vi "maxint_backup.vi"() -> ()   [LabVIEW 2020]
uses:
  <vilib>/userdefined/High Color/IMAQdx.ctl
  C:/Users/lenovo/source/repos/MSMQ_try/how/bin/Release/how.dll
  source/repos/MSMQ_try/how/bin/Release/how.dll
  C:/Users/lenovo/source/repos/MSMQ_try/Calculator/bin/Debug/Calculator.dll
  source/repos/MSMQ_try/Calculator/bin/Debug/Calculator.dll
  C:/Users/lenovo/source/repos/MSMQ_try/Pallete_maker/bin/Debug/Pallete_maker.dll
  source/repos/MSMQ_try/Pallete_maker/bin/Debug/Pallete_maker.dll
  C:/Users/lenovo/source/repos/MSMQ_try/MIrror_x64/bin/Debug/MIrror_x64.dll
  source/repos/MSMQ_try/MIrror_x64/bin/Debug/MIrror_x64.dll
  <vilib>/vision/driver/NI_Vision_Acquisition_Software.lvlib
  <resource>/objmgr/imaqdx.rc
  source/repos/cont2019/x64/Release/Image_processing.dll
panel:
  in  "log_data":i32=1
  in  "Exposure time":dbl=5000.0
  out "Waveform Chart":dbl(graph)
  in  "amplitude_limit":dbl=0.1
  in  "phi_v":dbl
  in  "phi_g":dbl=1.6
  in  "phi_p":dbl=1.2
  in  "vel_limit":dbl=0.4
  in  "init_zero":bool
  in  "level":dbl
  in  "factor":dbl
  out "Waveform Graph 2":dbl[](graph)
  in  "gamma":dbl=0.1
  in  "stop":bool
  in  "cam":bool
  out "mirror params":string
  in  "DM":bool
  out "Iterations":i32
  out "global_best_value":dbl
  out "Waveform Graph":dbl[](graph)
  out "Image":T1(plugin-control)
  out "metrics":dbl[](array[numeric])
  out "Numeric":dbl
  out "Exposure time":dbl
  out "najor":bool
  out "width":i32
  out "height":i32
  out "Intensity Graph":u8[][](graph)
  in  "Session In":T2="cam2"
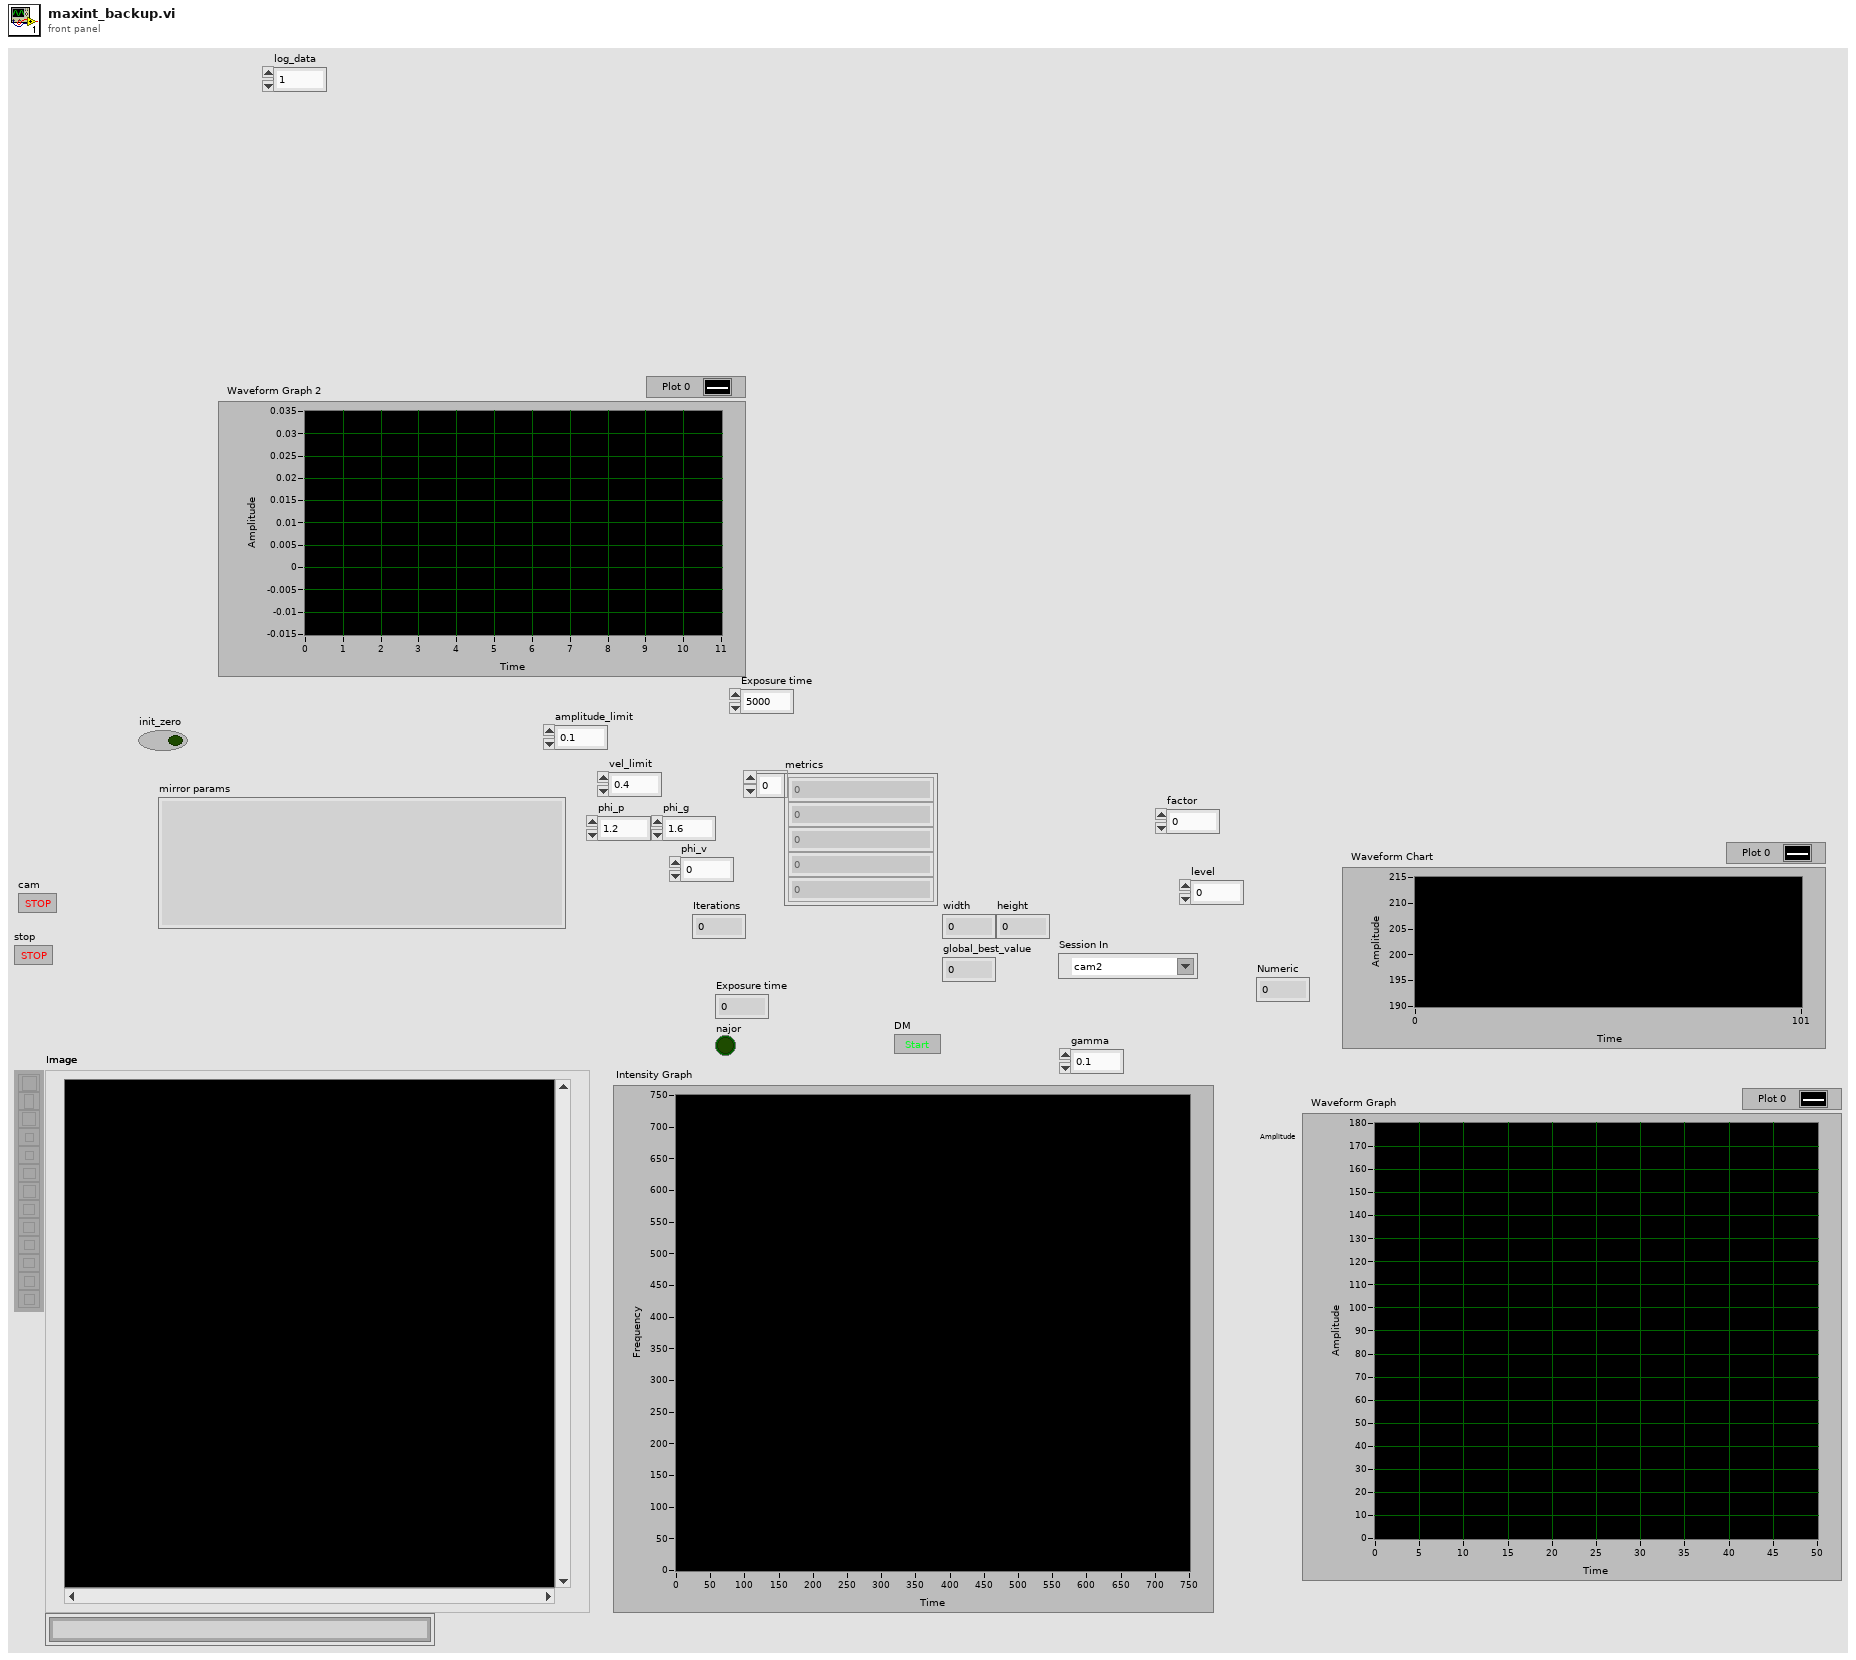
[diagram p1: front panel]
types:
  T1 = typedef "IMAQ Image.ctl" = refnum<image>
  T2 = typedef "IMAQdx.ctl" = refnum<k21>
  T3 = enum32{"Gray", "Binary", "Gradient", "Rainbow", "Temperature"}
  T4 = cluster{"Global Rectangle":i32[], "Contours":cluster{"Contour Type":u32, "ROI Type":u32, "Points":i32[]}[]}
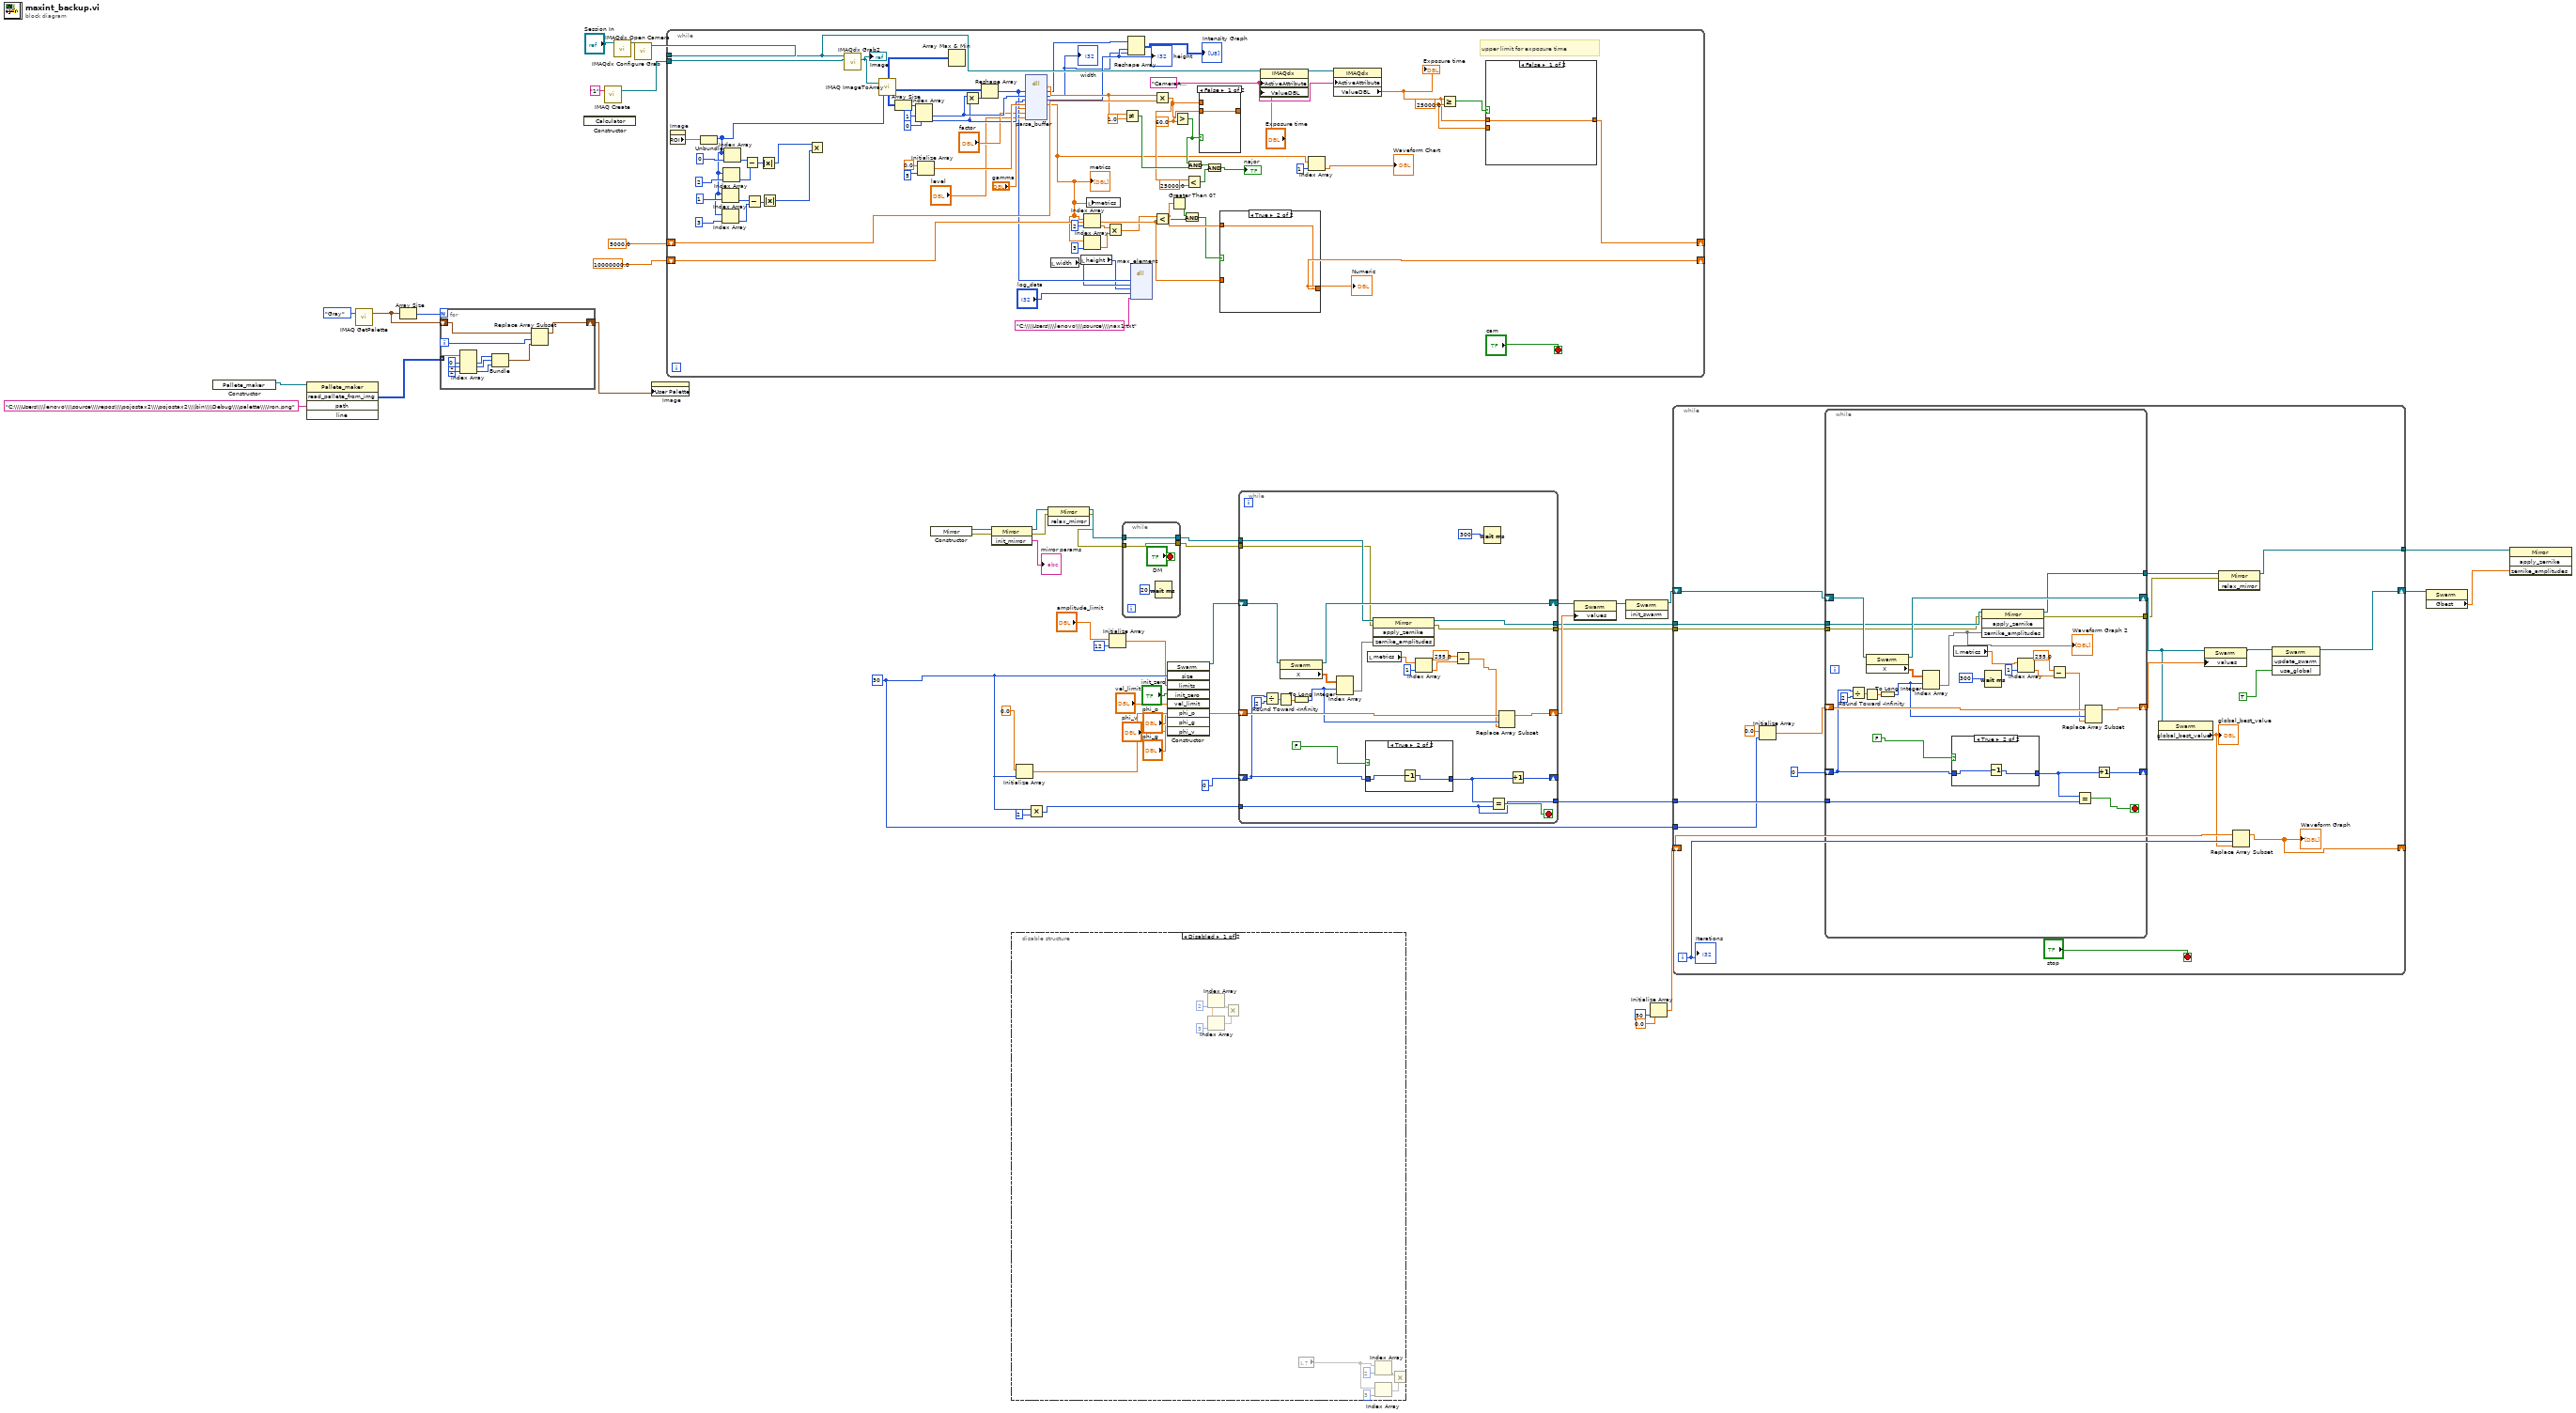
[diagram p0: block diagram]
diagram:
  w26 = 30 ("size")
  n1 = constructor class="Pallete_maker"() -> (reference out=w39:refnum<k24>)  [unwired: 3 in, 2 out]
  n2 = invoke class="Pallete_maker" method="read_pallete_from_img"(reference=w39, "path"="C:\\\\Users\\\\lenovo\\\\source\\\\repos\\\\pojostax2\\\\pojostax2\\\\bin\\\\Debug\\\\palette\\\\Iron.png") -> ("read_pallete_from_img"=w40:u8[][])  [unwired: 3 in, 4 out]
  n3 = call "IMAQ GetPalette"("Palette Number (gray)"=T3."Gray") -> ("Color Palette"=w42:cluster{"Red":u8, "Green":u8, "Blue":u8}[])  [unwired: 4 in, 1 out]
  n4 = Array Size(array=w42) -> (size(s)=w43:i32)
  n5 = for {
    N: w43 -> [_]
    shift-right: [w52] -> w38
    shift-left: w42 -> [w54]
    tunnel: w40 -> [w62] mode=indexing
    i -> [w53]
    n6 = Index Array(array=w62, index #1=0 ("index"), index #2=1 ("index"), index #3=2 ("index")) -> (element #1=w58:u8, element #2=w57:u8, element #3=w56:u8)
    n7 = Bundle(w58, w57, w56) -> (w55:cluster{u8, u8, u8})  [unwired: 1 in]
    n8 = Replace Array Subset(array=w54, new element=w55, index=w53) -> (w52:cluster{"Red":u8, "Green":u8, "Blue":u8}[])
  }
  n9 = constructor class="Calculator"() -> ()  [unwired: 3 in, 3 out]
  n10 = call "IMAQ Create"("Image Name"="1") -> ("New Image"=w47:T1)  [unwired: 4 in, 1 out]
  n11 = call <vilib>:"IMAQdx Open Camera.vi"("Session In"="Session In") -> ("Session Out"=w49:T2)  [unwired: 9 in, 1 out]
  n12 = call <vilib>:"IMAQdx Configure Grab.vi"("Session In"=w49) -> ("Session Out"=w48:T2)  [unwired: 9 in, 1 out]
  n13 = property on="Image" class="ImageControl"("User Palette"=w38) -> ()  [unwired: 2 in, 2 out]
  n14 = while {
    tunnel: w48 -> [w106]
    tunnel: w47 -> [w133]
    shift-right: [w112] -> _
    shift-left: 10000000.0 -> [w111]
    shift-right: [w101] -> _
    shift-left: 5000.0 -> [w100]
    stop <- "cam" stop-if-true
    w96 = 60.0 ("y")
    w102 = 25000.0 ("y")
    w104 = "CameraAttributes::AcquisitionControl::ExposureTime" ("ValueString")
    # "upper limit for exposure time"
    n15 = property on="Image" class="ImageControl"() -> ("ROI"=w132:T4)  [unwired: 2 in, 2 out]
    n16 = Unbundle(w132) -> ("Global Rectangle"=w121:i32[])  [unwired: 1 out]
    n17 = Index Array(array=w121, index=1) -> (element=w120:i32)
    n18 = Index Array(array=w121, index=3) -> (element=w119:i32)
    n19 = Index Array(array=w121, index=2) -> (element=w122:i32)
    n20 = Index Array(array=w121, index=0) -> (element=w123:i32)
    n21 = Subtract(x=w123, y=w122) -> (x-y=w118:i32)
    n22 = Subtract(x=w120, y=w119) -> (x-y=w117:i32)
    n23 = Absolute Value(x=w118) -> (abs(x)=w92:i32)
    n24 = Absolute Value(x=w117) -> (abs(x)=w93:i32)
    n25 = Multiply(x=w92, y=w93) -> ()  [unwired: 1 out]
    n26 = call <vilib>:"IMAQdx Grab2.vi"("Image In"=w133, "Session In"=w106) -> ("Image Out"=w128:T1)  [unwired: 6 in, 3 out]
    "Image" <- w128
    n27 = call "IMAQ ImageToArray"("Optional Rectangle"=w121, "Image"=w128) -> ("Image Pixels (U8)"=w91:u8[][])  [unwired: 2 in, 4 out]
    n28 = Array Size(array=w91) -> (size(s)=w90:i32[])
    n29 = Index Array(array=w90, index #1=1 ("index"), index #2=0 ("index")) -> (element #1=w86:i32, element #2=w85:i32)
    n30 = Initialize Array(0.0, 5 ("dimension size")) -> (w129:dbl[])
    n31 = Array Max & Min(array=w91) -> ()  [unwired: 4 out]
    n32 = Multiply(x=w86, y=w85) -> (x*y=w87:i32)
    n33 = Reshape Array(w91, w87) -> (w65:u8[])
    n34 = dll-call lib="C:/Users/lenovo/source/repos/cont2019/x64/Release/Image_processing.dll" fn="parse_buffer"("pixel_data"=w65, "width"=w86, "height"=w85, "metrics"=w129, "gamma"="gamma", "factor"="factor", "level"="level") -> ("ET_factor"=w98:dbl, "pixel_data"=w84:u8[], "width"=w82:i32, "height"=w83:i32, "metrics"=w71:dbl[])  [unwired: 6 in, 2 out]
    "metrics" <- w71
    "width" <- w82
    "height" <- w83
    n35 = local read "width"() -> (w64:i32)
    n36 = local read "height"() -> (w63:i32)
    n37 = Index Array(array=w71, index=2) -> (element=w115:dbl)
    n38 = Index Array(array=w71, index=3) -> (element=w116:dbl)
    n39 = local write "metrics"(w71) -> ()
    n40 = Multiply(x=w115, y=w116) -> (x*y=w110:dbl)
    n41 = Not Equal?(x=w98, y=1.0) -> (x != y?=w95:bool)
    n42 = Reshape Array(w84, w83, w82) -> (→"Intensity Graph":u8[][])
    n43 = dll-call lib="C:/Users/lenovo/source/repos/cont2019/x64/Release/Image_processing.dll" fn="max_element"("pixel_data"=w65, "width"=w64, "height"=w63, "log_data"="log_data", "path"="C:\\\\Users\\\\lenovo\\\\source\\\\nax1.txt") -> ()  [unwired: 9 in, 2 out]
    n44 = Multiply(x=w98, y=w100) -> (x*y=w78:dbl)
    n45 = Less?(x=w110, y=w111) -> (x < y?=w108:bool)
    n46 = Greater Than 0?(x=w110) -> (x > 0?=w109:bool)
    n47 = Greater?(x=w78, y=w96) -> (0:w94:bool)
    n48 = And(x=w109, y=w108) -> (x .and. y?=w107:bool)
    n49 = Less?(x=w78, y=25000.0) -> (x < y?=w81:bool)
    n50 = And(x=w94, y=w95) -> (x .and. y?=w80:bool)
    n51 = case shown="False" w94 {
      tunnel: [w134 w135] -> _
      tunnel: w78 -> [_ w135]
      tunnel: w96 -> [w134 _]
      frame False {
      }
      frame True {
      }
    }
    n52 = And(x=w80, y=w81) -> (x .and. y?=→"najor":bool)
    n53 = case shown="True" w107 {
      tunnel: [w138 w139] -> w112
      tunnel: w111 -> [w138 _]
      tunnel: w110 -> [_ w139]
      frame False {
      }
      frame True {
      }
    }
    "Numeric" <- w112
    n54 = property class="IMAQdx"(reference=w106, "ActiveAttribute"=w104, "ValueDBL"="Exposure time") -> (reference out=w105:T2)  [unwired: 1 in, 1 out]
    n55 = Index Array(array=w71, index=1) -> (element=→"Waveform Chart":dbl)
    n56 = property class="IMAQdx"(reference=w105, "ActiveAttribute"=w104) -> ("ValueDBL"=w99:dbl)  [unwired: 1 in, 2 out]
    "Exposure time" <- w99
    n57 = Greater Or Equal?(x=w99, y=w102) -> (x >= y?=w103:bool)
    n58 = case shown="False" w103 {
      tunnel: w102 -> [_ w137]
      tunnel: [w136 w137] -> w101
      tunnel: w99 -> [w136 _]
      frame False {
      }
      frame True {
      }
    }
  }
  n59 = constructor class="Mirror"() -> (reference out=w22:refnum<k24>, error out=w20:errorcluster)  [unwired: 3 in, 1 out]
  n60 = invoke class="Mirror" method="init_mirror"(reference=w22, error in=w20) -> (reference out=w15:refnum<k24>, error out=w14:errorcluster, "init_mirror"=→"mirror params":string)  [unwired: 1 in]
  n61 = disable-structure shown="Disabled" {
    frame Disabled {
      n62 = Index Array(index=3) -> (array=w140:dbl[], element=w144)
      n63 = Index Array(array=w140, index=2) -> (element=w143)
      n64 = Multiply(x=w143, y=w144) -> ()  [unwired: 1 out]
      n65 = local read item#-1() -> (w145)
      n66 = Index Array(array=w145, index=2) -> (element=w148)
      n67 = Index Array(array=w145, index=3) -> (element=w149)
      n68 = Multiply(x=w148, y=w149) -> ()  [unwired: 1 out]
    }
    frame Enabled {
    }
  }
  n69 = Initialize Array(0.0 ("element"), w26) -> (w34:dbl[])
  n70 = Multiply(x=w26, y=2) -> (x*y=w29:i32)
  n71 = invoke class="Mirror" method="relax_mirror"(reference=w15, error in=w14) -> (reference out=w13:refnum<k24>, error out=w12:errorcluster)  [unwired: 1 in, 1 out]
  n72 = Initialize Array("amplitude_limit", 12 ("dimension size")) -> (w4:dbl[])
  n73 = while {
    tunnel: [w152] -> w19
    tunnel: w13 -> [w152]
    tunnel: [w150] -> w18
    tunnel: w12 -> [w150]
    stop <- "DM" stop-if-true
    n74 = Wait (ms)(milliseconds to wait=u32 20) -> ()  [unwired: 1 out]
  }
  n75 = constructor class="Swarm"("size"=w26, "limits"=w4, "init_zero"="init_zero", "vel_limit"="vel_limit", "phi_p"="phi_p", "phi_g"="phi_g", "phi_v"="phi_v") -> (reference out=w35:refnum<k24>)  [unwired: 3 in, 9 out]
  n76 = while {
    shift-right: [w172] -> w32
    shift-left: w34 -> [w173]
    shift-right: [w170] -> w33
    shift-left: w35 -> [w179]
    shift-right: [w169] -> _
    shift-left: 0 -> [w167]
    tunnel: w29 -> [w165]
    tunnel: [w165] -> w27
    tunnel: w19 -> [w164]
    tunnel: w18 -> [w162]
    tunnel: [w161] -> w17
    tunnel: [w160] -> w16
    stop <- w168 stop-if-true
    n77 = Divide(x=w167, y=2) -> (x/y=w177:dbl)
    n78 = Round Toward -Infinity(1:w177) -> (0:w176:dbl)
    n79 = property class="Swarm"(reference=w179) -> (reference out=w170:refnum<k24>, "X"=w175:dbl[][])  [unwired: 1 in, 1 out]
    n80 = To Long Integer(number=w176) -> (32bit integer=w171:i32)
    n81 = Index Array(array=w175, index (row)=w171) -> (element=w163:dbl[])  [unwired: 1 in]
    n82 = case shown="True" FALSE {
      tunnel: w167 -> [w180 w182]
      tunnel: [w180 w181] -> w166
      frame False {
      }
      frame True {
        n83 = Decrement(x=w182) -> (x-1=w181:i32)
      }
    }
    n84 = local read "metrics"() -> (w159:dbl[])
    n85 = invoke class="Mirror" method="apply_zernike"(reference=w164, error in=w162, "zernike_amplitudes"=w163) -> (reference out=w161:refnum<k24>, error out=w160:errorcluster)  [unwired: 1 in, 2 out]
    n86 = Index Array(array=w159, index=1) -> (element=w157:dbl)
    n87 = Subtract(x=255.0, y=w157) -> (x-y=w155:dbl)
    n88 = Wait (ms)(milliseconds to wait=u32 300) -> ()  [unwired: 1 out]
    n89 = Equal?(x=w166, y=w165) -> (x = y?=w168:bool)
    n90 = Replace Array Subset(array=w173, new element=w155, index=w171) -> (w172:dbl[])
    n91 = Increment(x=w166) -> (x+1=w169:i32)
  }
  n92 = property class="Swarm"(reference=w33, "values"=w32) -> (reference out=w31:refnum<k24>)  [unwired: 1 in, 1 out]
  n93 = invoke class="Swarm" method="init_swarm"(reference=w31) -> (reference out=w28:refnum<k24>)  [unwired: 2 in, 2 out]
  n94 = Initialize Array(0.0 ("element"), 50 ("dimension size")) -> (w23:dbl[])
  n95 = while {
    tunnel: w27 -> [w201]
    tunnel: w26 -> [w200]
    shift-right: [w194] -> w2
    shift-left: w28 -> [w203]
    shift-right: [w189] -> _
    shift-left: w23 -> [w192]
    tunnel: w17 -> [w188]
    tunnel: w16 -> [w187]
    tunnel: [w183] -> w3
    i -> [w191]
    stop <- "stop" stop-if-true
    n96 = Initialize Array(0.0 ("element"), w200) -> (w198:dbl[])
    n97 = while {
      shift-right: [w222] -> w197
      shift-left: w198 -> [w223]
      shift-right: [w220] -> w193
      shift-left: w203 -> [w229]
      shift-right: [w219] -> _
      shift-left: 0 -> [w217]
      tunnel: w201 -> [w218]
      tunnel: w188 -> [w215]
      tunnel: w187 -> [w214]
      tunnel: [w213] -> w186
      tunnel: [w212] -> w185
      stop <- w211 stop-if-true
      n98 = Divide(x=w217, y=2) -> (x/y=w227:dbl)
      n99 = Round Toward -Infinity(1:w227) -> (0:w226:dbl)
      n100 = property class="Swarm"(reference=w229) -> (reference out=w220:refnum<k24>, "X"=w225:dbl[][])  [unwired: 1 in, 1 out]
      n101 = To Long Integer(number=w226) -> (32bit integer=w221:i32)
      n102 = Index Array(array=w225, index (row)=w221) -> (element=w210:dbl[])  [unwired: 1 in]
      "Waveform Graph 2" <- w210
      n103 = case shown="True" FALSE {
        tunnel: w217 -> [w230 w232]
        tunnel: [w230 w231] -> w216
        frame False {
        }
        frame True {
          n104 = Decrement(x=w232) -> (x-1=w231:i32)
        }
      }
      n105 = local read "metrics"() -> (w209:dbl[])
      n106 = invoke class="Mirror" method="apply_zernike"(reference=w215, error in=w214, "zernike_amplitudes"=w210) -> (reference out=w213:refnum<k24>, error out=w212:errorcluster)  [unwired: 1 in, 2 out]
      n107 = Wait (ms)(milliseconds to wait=u32 300) -> ()  [unwired: 1 out]
      n108 = Index Array(array=w209, index=1) -> (element=w207:dbl)
      n109 = Subtract(x=255.0, y=w207) -> (x-y=w205:dbl)
      n110 = Equal?(x=w216, y=w218) -> (x = y?=w211:bool)
      n111 = Replace Array Subset(array=w223, new element=w205, index=w221) -> (w222:dbl[])
      n112 = Increment(x=w216) -> (x+1=w219:i32)
    }
    n113 = property class="Swarm"(reference=w193) -> ("global_best_value"=w190:dbl)  [unwired: 1 in, 2 out]
    "global_best_value" <- w190
    n114 = property class="Swarm"(reference=w193, "values"=w197) -> (reference out=w196:refnum<k24>)  [unwired: 1 in, 1 out]
    n115 = invoke class="Mirror" method="relax_mirror"(reference=w186, error in=w185) -> (reference out=w183:refnum<k24>)  [unwired: 1 in, 2 out]
    n116 = Replace Array Subset(array=w192, new element=w190, index=w191) -> (w189:dbl[])
    "Waveform Graph" <- w189
    n117 = invoke class="Swarm" method="update_swarm"(reference=w196, "use_global"=TRUE) -> (reference out=w194:refnum<k24>)  [unwired: 2 in, 3 out]
    "Iterations" <- w191
  }
  n118 = property class="Swarm"(reference=w2) -> ("Gbest"=w1:dbl[])  [unwired: 1 in, 2 out]
  n119 = invoke class="Mirror" method="apply_zernike"(reference=w3, "zernike_amplitudes"=w1) -> ()  [unwired: 2 in, 4 out]
